vi "QMH_Template.vi"   [LabVIEW 2025]
uses:
  <vilib>/Handler Framework/Handler Framework.lvlib
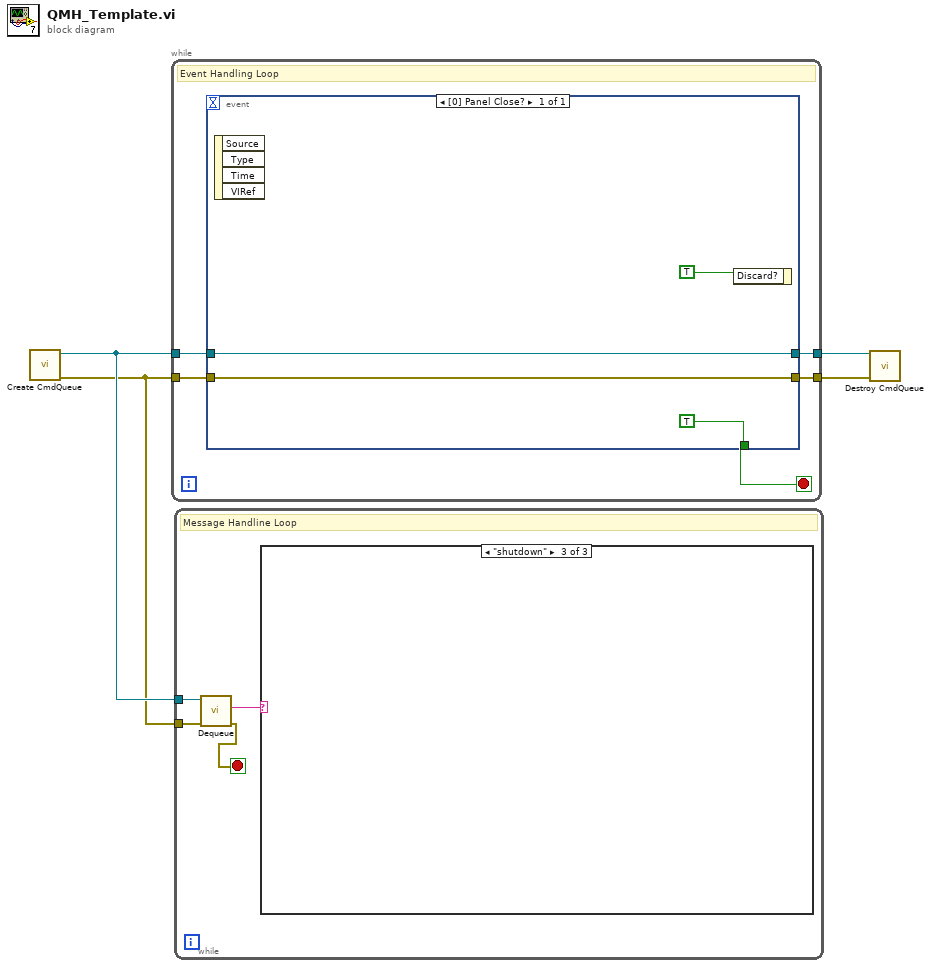
[diagram p0: block diagram]
diagram:
  n1 = call <vilib>:"Create CmdQueue.vi"() -> ("error out"=w3:errorcluster, "CmdQueue out"=w4:refnum<queue>)  [unwired: 10 in]
  n2 = while {
    tunnel: w4 -> [w8]
    tunnel: w3 -> [w7]
    tunnel: [w6] -> w2
    tunnel: [w5] -> w1
    stop <- w9 stop-if-true
    # "Event Handling Loop"
    n3 = event shown="[0] Panel Close?" {
      selector: _ -> [_]
      dyn-events: _ -> [_]
      timeout: _ -> [_]
      tunnel: [TRUE] -> w9
      tunnel: w8 -> [w11]
      tunnel: w7 -> [w10]
      tunnel: [w11] -> w6
      tunnel: [w10] -> w5
      event Panel Close? {
        n4 = event-data() -> ()  [unwired: 1 in, 4 out]
        n5 = event-data("Discard?"=TRUE) -> ()  [unwired: 1 in, 1 out]
      }
    }
  }
  n6 = while {
    tunnel: w4 -> [w17]
    tunnel: w3 -> [w16]
    stop <- w15 stop-if-true
    # "Message Handline Loop"
    n7 = call <vilib>:"Dequeue.vi"("error in (no error)"=w16, "CmdQueue in"=w17) -> ("error out"=w15:errorcluster, "cmd"=w14:string)  [unwired: 5 in, 3 out]
    n8 = case shown="\"shutdown\"" w14 {
      frame Default {
      }
      frame "init" {
      }
      frame "shutdown" {
      }
    }
  }
  n9 = call <vilib>:"Destroy CmdQueue.vi"("error in (no error)"=w1, "CmdQueue in"=w2) -> ()  [unwired: 9 in, 1 out]
